vi "_Get File.vi"(4 "For Write (T)":bool=TRUE, 5 "select mode (new or existing)":T1(ring)=enum."new or existing file", 6 "default name":string="My Data.isd", 7 "extension (isd)":string="*.isd", 8 "prompt":string="Please enter a data file name.", 9 "Start Path":path) -> (0 "cancelled":bool, 1 "Seleted File":path, 2 "Exists":bool, 3 "Succeeded":bool)   [LabVIEW 2015]
doc: "Obtain a file name."
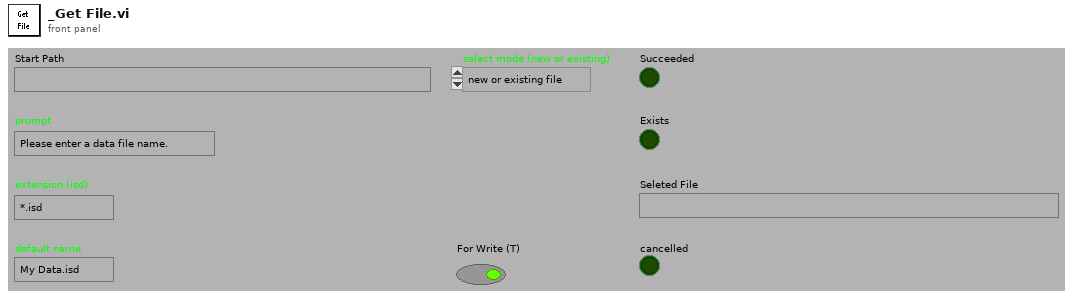
[diagram p1: front panel]
types:
  T1 = enum32{"existing file", "new file", "new or existing file", "existing dir", "new dir", "new or existing dir", "existing file (use LLBs)", "new file (use LLBs)", "new or existing file (use LLBs)", "new or existing file or directory (use LLBs)"}
  T2 = enum16{"Left Button", "Center Button", "Right Button", "Window Close"}
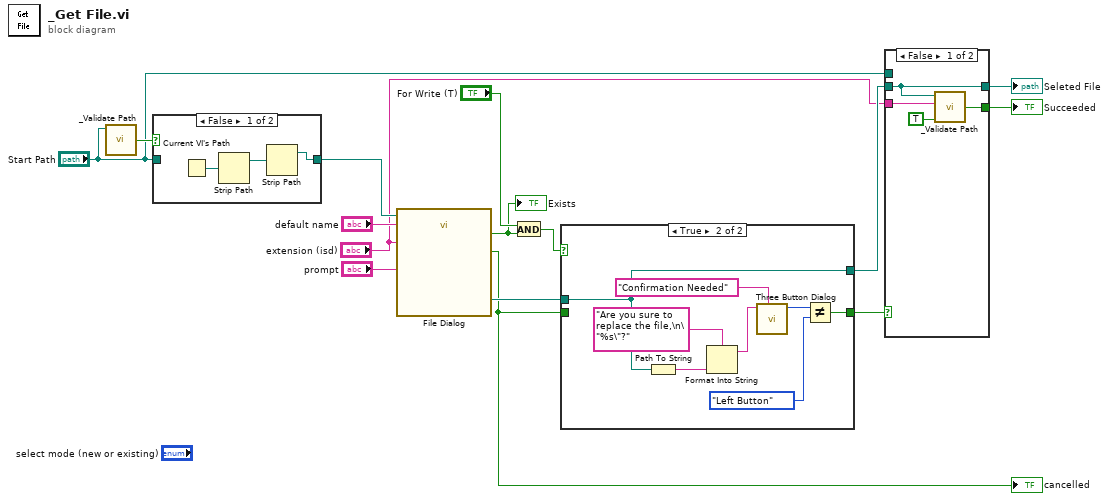
[diagram p0: block diagram]
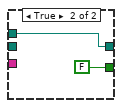
[diagram p3: hidden frame]
diagram:
  n1 = call "_Validate Path.vi"("path"="Start Path") -> ("Valid"=w15:bool)  [unwired: 3 in]
  n2 = case shown="False" w15 {
    tunnel: "Start Path" -> [_ w19]
    tunnel: [w16 w19] -> w5
    frame False {
      n3 = Current VI's Path() -> (path=w18:path)
      n4 = Strip Path(path=w18) -> (stripped path=w17:path)  [unwired: 1 out]
      n5 = Strip Path(path=w17) -> (stripped path=w16:path)  [unwired: 1 out]
    }
    frame True {
    }
  }
  n6 = call "File Dialog"("start path"=w5, "prompt"="prompt", "default name"="default name", "pattern (all files)"="extension (isd)") -> ("selected path"=w3:path, "exists"=w2:bool, "cancelled"=w1:bool)  [unwired: 8 in, 1 out]
  "Exists" <- w2
  "cancelled" <- w1
  n7 = And(x="For Write (T)", y=w2) -> (x .and. y?=w10:bool)
  n8 = case shown="True" w10 {
    tunnel: w3 -> [w21 w22]
    tunnel: [w21 w22] -> w9
    tunnel: w1 -> [w20 _]
    tunnel: [w20 w23] -> w8
    frame False {
    }
    frame True {
      n9 = Path To String(path=w22) -> (string=w29:string)
      n10 = Format Into String(format string="Are you sure to replace the file,\n\"%s\"?", w29) -> (resulting string=w27:string)  [unwired: 2 in, 1 out]
      n11 = call <vilib>:"Three Button Dialog.vi"("Window Title (\"\")"="Confirmation Needed", "message"=w27) -> ("Which Button?"=w25:T2)  [unwired: 3 in, 6 out]
      n12 = Not Equal?(x=w25, y=T2."Left Button") -> (x != y?=w23:bool)
    }
  }
  n13 = case shown="False" w8 {
    tunnel: [w33 w35] -> w13
    tunnel: "Start Path" -> [_ w35]
    tunnel: w9 -> [w33 _]
    tunnel: [w32 FALSE ("Valid")] -> w12
    tunnel: "extension (isd)" -> [w31 _]
    frame False {
      n14 = call "_Validate Path.vi"("Check Type (F)"=TRUE ("Check Exist"), "Type (isd)"=w31, "path"=w33) -> ("Valid"=w32:bool)  [unwired: 1 in]
    }
    frame True {
    }
  }
  "Seleted File" <- w13
  "Succeeded" <- w12
